vi "Data_PSD.vi"() -> ()   [LabVIEW 2020]
doc: "Use this template to build a producer/consumer design pattern. Use this template when you need to execute a process, such as data analysis, when a data source, such as a triggered acquisition, produces data at an uneven rate and you need to execute the process when the data becomes available."
uses:
  <vilib>/Utility/error.llb/DialogType.ctl
  <vilib>/measure/maspectr.llb/Power Spectrum and PSD Export Mode.ctl
  <vilib>/measure/maspectr.llb/FFT Power Spectrum and PSD for 1 Chan.vi
  <vilib>/Analysis/0measdsp.llb/Scaled Time Domain Window (DBL).vi
  <vilib>/sound2/lvsound2.llb/Sound File Info (path).vi
  <vilib>/sound2/lvsound2.llb/Sound File Read Open.vi
  <vilib>/sound2/lvsound2.llb/Sound File Read (DBL).vi
  <vilib>/Analysis/NI_AALPro.lvlib
  <vilib>/measure/NI_MAPro.lvlib
panel:
  out "Signal":waveform(dbl)(graph)
  out "Max Amplitude":dbl
  out "PSD of Signal":cluster{"f0":dbl, "df":dbl, "S(f)":dbl[]}(graph)
  out "total number of samples/ch":u32
  in  "Path wav":path
  out "Frequency Peak":dbl format="%0.4f"
  in  "stop":bool
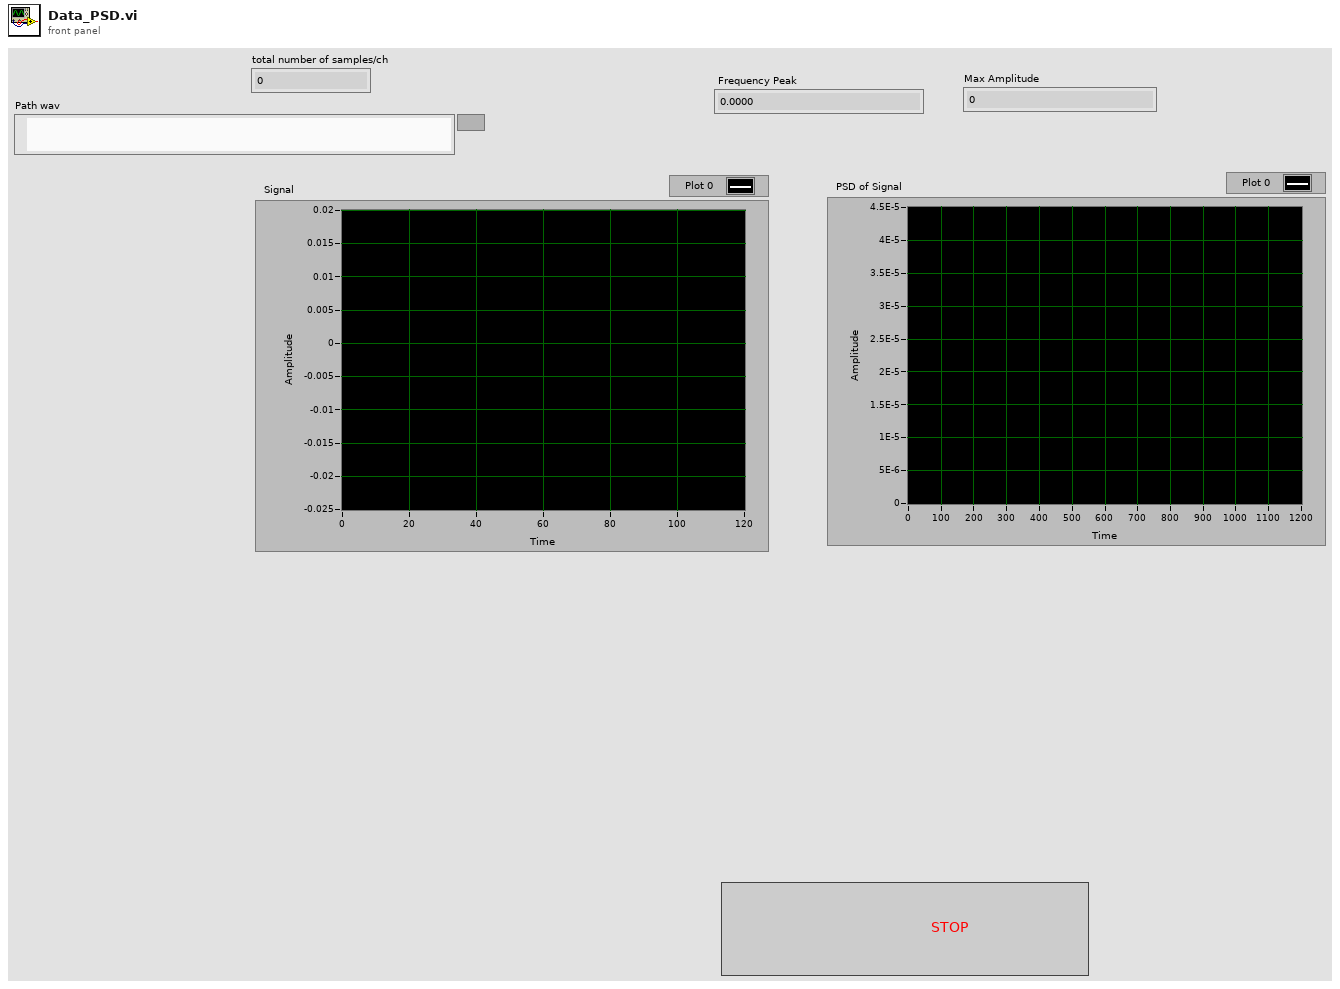
[diagram p1: front panel]
types:
  T1 = typedef "DialogType.ctl" = u16
  T2 = typedef "NI_MAPro.lvlib/Power Spectrum and PSD Export Mode.ctl" = u16
  T3 = typedef "Sound File Refnum.ctl" = refnum<file>
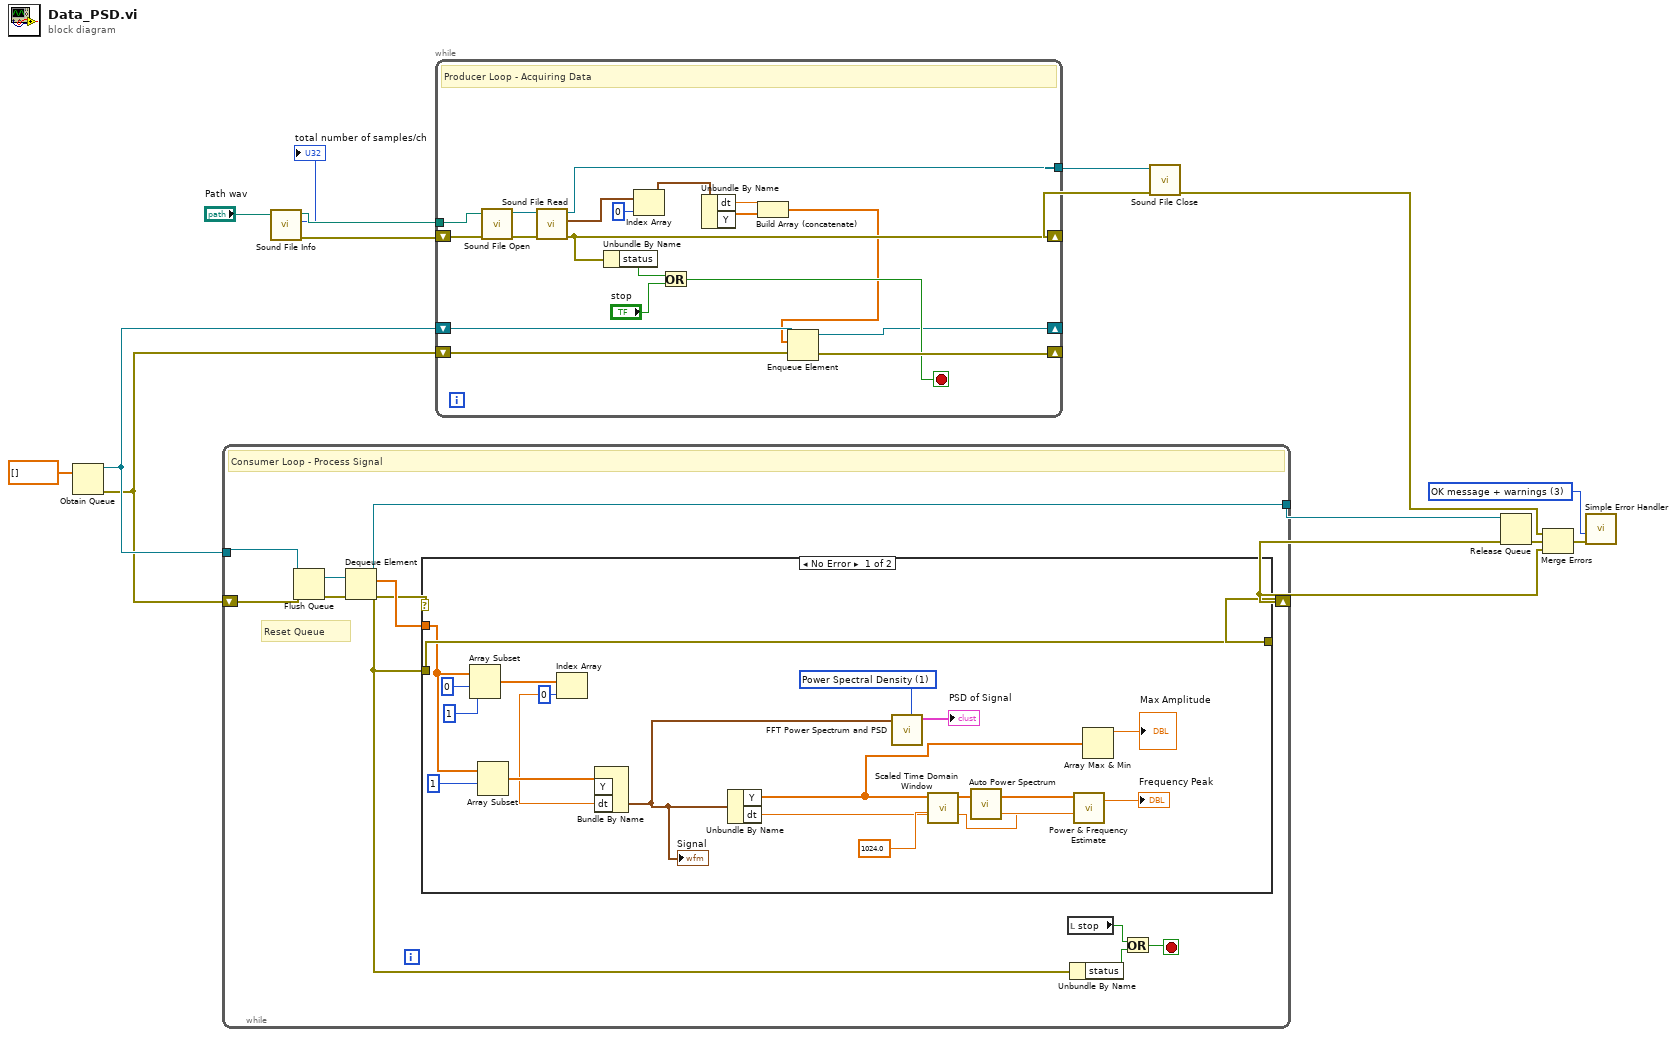
[diagram p0: block diagram]
diagram:
  w14 = T1 3 items=["no dialog", "OK message", "continue or stop message", "OK message + warnings", "continue/stop + warnings"] ("type of dialog (OK msg:1)")
  n1 = Obtain Queue(element data type=dbl[] []) -> (queue out=w15:refnum<queue>, error out=w12:errorcluster)  [unwired: 3 in, 2 out]
  n2 = while {
    tunnel: w15 -> [w21]
    shift-right: [w26] -> w9
    shift-left: w12 -> [w19]
    tunnel: [w17] -> w10
    stop <- w22 stop-if-true
    # "Reset Queue"
    # "Consumer Loop - Process Signal"
    n3 = Flush Queue(queue=w21, error in (no error)=w19) -> (queue out=w20:refnum<queue>, error out=w18:errorcluster)  [unwired: 1 out]
    n4 = Dequeue Element(queue=w20, error in (no error)=w18) -> (queue out=w17:refnum<queue>, element=w25:dbl[], error out=w16:errorcluster)  [unwired: 2 out]
    n5 = case shown="No Error" w16 {
      tunnel: w25 -> [w37 _]
      tunnel: [w42 w47] -> w26
      tunnel: w16 -> [w42 w47]
      frame No Error {
        w40 = T2 1 items=["Power Spectrum", "Power Spectral Density"] ("export mode")
        n6 = Array Subset(array=w37, index=0, length=1) -> (w35:dbl[])
        n7 = Array Subset(array=w37, index=1) -> (w36:dbl[])  [unwired: 1 in]
        n8 = Index Array(array=w35, index=0) -> (element=w33:dbl)
        n9 = Bundle By Name("Y"=w36, "dt"=w33) -> (w28:waveform(dbl))  [unwired: 1 in]
        "Signal" <- w28
        n10 = Unbundle By Name(w28) -> ("Y"=w27:dbl[], "dt"=w39:dbl)
        n11 = call-poly <vilib>:"FFT Power Spectrum and PSD.vi"("export mode"=w40, "time signal"=w28) -> ("Power Spectrum / PSD"=→"PSD of Signal":cluster{"f0":dbl, "df":dbl, "magnitude":dbl[]})  [unwired: 6 in, 3 out]
        n12 = call-poly <vilib>:"Scaled Time Domain Window.vi"("window parameter"=1024.0, "X"=w27) -> ("Windowed X"=w44:dbl[])  [unwired: 1 in, 8 out]
        n13 = call <vilib>:"Auto Power Spectrum.vi"("dt"=w39, "Signal (V)"=w44) -> ("df"=w45:dbl, "Power Spectrum (V^2 rms)"=w30:dbl[])
        n14 = call <vilib>:"Power & Frequency Estimate.vi"("df"=w45, "Power Spectrum (V^2 rms)"=w30) -> ("est frequency peak"=→"Frequency Peak":dbl)  [unwired: 3 in, 2 out]
        n15 = Array Max & Min(array=w27) -> (max value=→"Max Amplitude":dbl)  [unwired: 3 out]
      }
      frame Error {
      }
    }
    n16 = local read "stop"() -> (w24:bool)
    n17 = Unbundle By Name(w16) -> ("status"=w23:bool)
    n18 = Or(x=w24, y=w23) -> (x .or. y?=w22:bool)
  }
  n19 = call-poly <vilib>:"Sound File Info.vi"("path"="Path wav") -> ("error out"=w6:errorcluster, "total number of samples/ch"=→"total number of samples/ch":u32, "path out"=w7:path)  [unwired: 7 in, 1 out]
  n20 = while {
    shift-right: [w64] -> _
    shift-left: w12 -> [w65]
    shift-right: [w51] -> _
    shift-left: w15 -> [w66]
    shift-right: [w52] -> w4
    shift-left: w6 -> [w58]
    tunnel: w7 -> [w60]
    tunnel: [w56] -> w5
    stop <- w61 stop-if-true
    # "Producer Loop - Acquiring Data"
    n21 = call-poly <vilib>:"Sound File Open.vi"("error in (no error)"=w58, "path"=w60) -> ("error out"=w57:errorcluster, "sound file refnum"=w59:T3)  [unwired: 8 in]
    n22 = call-poly <vilib>:"Sound File Read.vi"("error in (no error)"=w57, "sound file refnum"=w59) -> ("error out"=w52:errorcluster, "data"=w55:waveform(dbl)[], "sound file refnum out"=w56:T3)  [unwired: 5 in, 2 out]
    n23 = Unbundle By Name(w52) -> ("status"=w63:bool)
    n24 = Index Array(array=w55, index=0) -> (element=w53:waveform(dbl))
    n25 = Or(x=w63, y="stop") -> (x .or. y?=w61:bool)
    n26 = Unbundle By Name(w53) -> ("dt"=w50:dbl, "Y"=w49:dbl[])
    n27 = Build Array (concatenate)(w50, w49) -> (w48:dbl[])
    n28 = Enqueue Element(queue=w66, element=w48, error in (no error)=w65) -> (queue out=w51:refnum<queue>, error out=w64:errorcluster)  [unwired: 2 out]
  }
  n29 = call <vilib>:"Sound File Close.vi"("error in (no error)"=w4, "sound file refnum"=w5) -> ("error out"=w3:errorcluster)  [unwired: 9 in]
  n30 = Release Queue(queue=w10, error in (no error)=w9) -> (error out=w8:errorcluster)  [unwired: 1 in, 2 out]
  n31 = Merge Errors(w3, w8, w9) -> (w13:errorcluster)
  n32 = call <vilib>:"Simple Error Handler.vi"("type of dialog (OK msg:1)"=w14, "error in (no error)"=w13) -> ()  [unwired: 8 out]
